vi "Passed.vi"(11 "IO":T1) -> (3 "Node":refnum<class "bt_Node.lvclass">)   [LabVIEW 2021, in "Test Sequencer Support.lvlib"]
uses:
  Test Sequencer Support.lvlib
  IO Type.ctl
  <vilib>/TSA/Event Log/Event_TextLog/Event_TextLog.lvclass
  C:/Program Files (x86)/National Instruments/LabVIEW 2021/vi.lib/TSA/Event Log/abs_EventLog/abs_EventLog.lvclass
  Blackboard/Blackboard.lvclass
  <vilib>/TSA/Abstract Data Classes/Abs_Types/Boolean/Abs_Boolean.lvclass
  C:/Program Files (x86)/National Instruments/LabVIEW 2021/vi.lib/TSA/Abstract Data Classes/Abs_Types/Value/Abs_Value.lvclass
  <vilib>/TSA/Abstract Data Classes/Abs_Types/Waveform/Abs_Waveform.lvclass
  <vilib>/TSA/Abstract Data Classes/Abs_Types/Double Float/Abs_Double Float.lvclass
  Support/Nodes/abs_Node/bt_Node.lvclass
  Support/Nodes/Leaves/Log/bt_Log.lvclass
  C:/Users/timst/Documents/Repositories/LV_Behaviour_Tree/Source/Support/Nodes/abs_Node/bt_Node.lvclass
  <vilib>/TSA/Abstract Data Classes/Constants/Support/Str/Str.vi
  Support/Poly/Log/Log_StringClass.vi
  <vilib>/TSA/Abstract Data Classes/Constants/Support/Bool/Bool.vi
  <vilib>/TSA/Abstract Data Classes/Constants/Support/Str/Const_Str.lvclass
  BT.lvlib
  <vilib>/TSA/Abstract Data Classes/Constants/Support/Bool/Const_Bool.lvclass
  C:/Program Files (x86)/National Instruments/LabVIEW 2021/vi.lib/TSA/Event Log/Event_TextLog/Event_TextLog.lvclass
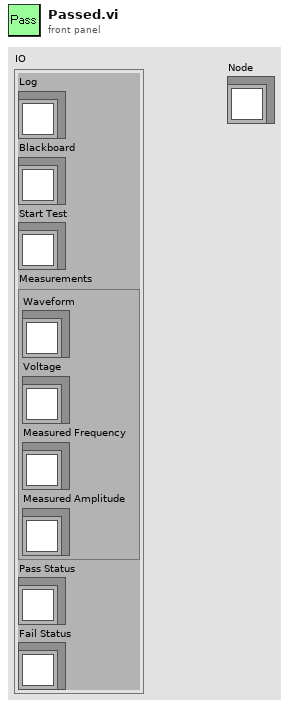
[diagram p1: front panel]
types:
  T1 = typedef "Test Sequencer Support.lvlib/IO Type.ctl" = cluster{"Log":refnum<class "Event_TextLog.lvclass">, "Blackboard":refnum<class "Blackboard.lvclass">, "Start Test":refnum<class "Abs_Boolean.lvclass">, "Measurements":cluster{"Waveform":refnum<class "Abs_Waveform.lvclass">, "Voltage":refnum<class "Abs_Double Float.lvclass">, "Measured Frequency":refnum<class "Abs_Double Float.lvclass">, "Measured Amplitude":refnum<class "Abs_Double Float.lvclass">}, "Pass Status":refnum<class "Abs_Boolean.lvclass">, "Fail Status":refnum<class "Abs_Boolean.lvclass">}
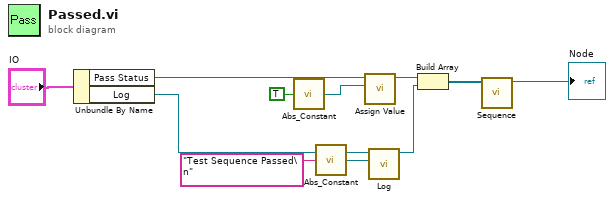
[diagram p0: block diagram]
diagram:
  n1 = Unbundle By Name("IO") -> ("Pass Status"=w1:refnum<class "Abs_Boolean.lvclass">, "Log"=w9:refnum<class "Event_TextLog.lvclass">)
  n2 = call-poly <vilib>:"Abs_Constant.vi"("Boolean"=TRUE) -> ("Abs_Boolean.lvclass"=w6:refnum<class "Abs_Boolean.lvclass">)  [unwired: 4 in]
  n3 = call-poly <vilib>:"Abs_Constant.vi"("String"="Test Sequence Passed\n") -> ("Abs_String.lvclass"=w11:refnum<class "Abs_String.lvclass">)  [unwired: 4 in]
  n4 = call "Assign Value.vi"("Assigned Value"=w6, "Value"=w1) -> ("Node Out"=w3:refnum<class "bt_Node.lvclass">)  [unwired: 9 in]
  n5 = call-poly "Log.vi"("Message"=w11, "EventLog"=w9) -> ("node out"=w4:refnum<class "bt_Log.lvclass">)  [unwired: 9 in]
  n6 = Build Array(w3, w4) -> (w7:refnum<class "bt_Node.lvclass">[])
  n7 = call "Sequence.vi"("Nodes"=w7) -> ("Node"=→"Node":refnum<class "bt_Node.lvclass">)  [unwired: 10 in]
